vi "Kernel grid search.vi"(8 "Error In":errorcluster, 10 "Grid parameters":T8={"C start"=-5.0, "Gamma start"=-15.0, "C end"=15.0, "C step"=4.0, "K"=10, "Gamma end"=3.0, "Gamma step"=4.0, "random seed"=-1}, 11 "Problem":T1) -> (0 "Error Out":errorcluster, 1 "Kernel":T6, 2 "libsvm":T5, 3 "3D Surface Plot":refnum<class "3D Plot Datatype.lvclass">[](array[class]), 4 "Grid search results":T2)   [LabVIEW 2016]
uses:
  <userlib>/LVLibSVM/LibSVM Sparse/Controls/Grid parameters.ctl
  <userlib>/LVLibSVM/LibSVM Sparse/Controls/Kernel.ctl
  <userlib>/LVLibSVM/LibSVM Sparse/Wrapper API/Controls/svm_kernel_type.ctl
  <userlib>/LVLibSVM/LibSVM Sparse/Controls/Options Training.ctl
  <userlib>/LVLibSVM/LibSVM Sparse/Controls/Parameters C_SVC.ctl
  <vilib>/Math Plots/3D Math Plots/3D Plot/3D Plot Datatype/3D Plot Datatype.lvclass
  <userlib>/LVLibSVM/LibSVM Dense/Wrapper API/Controls/svmdense_problem.ctl
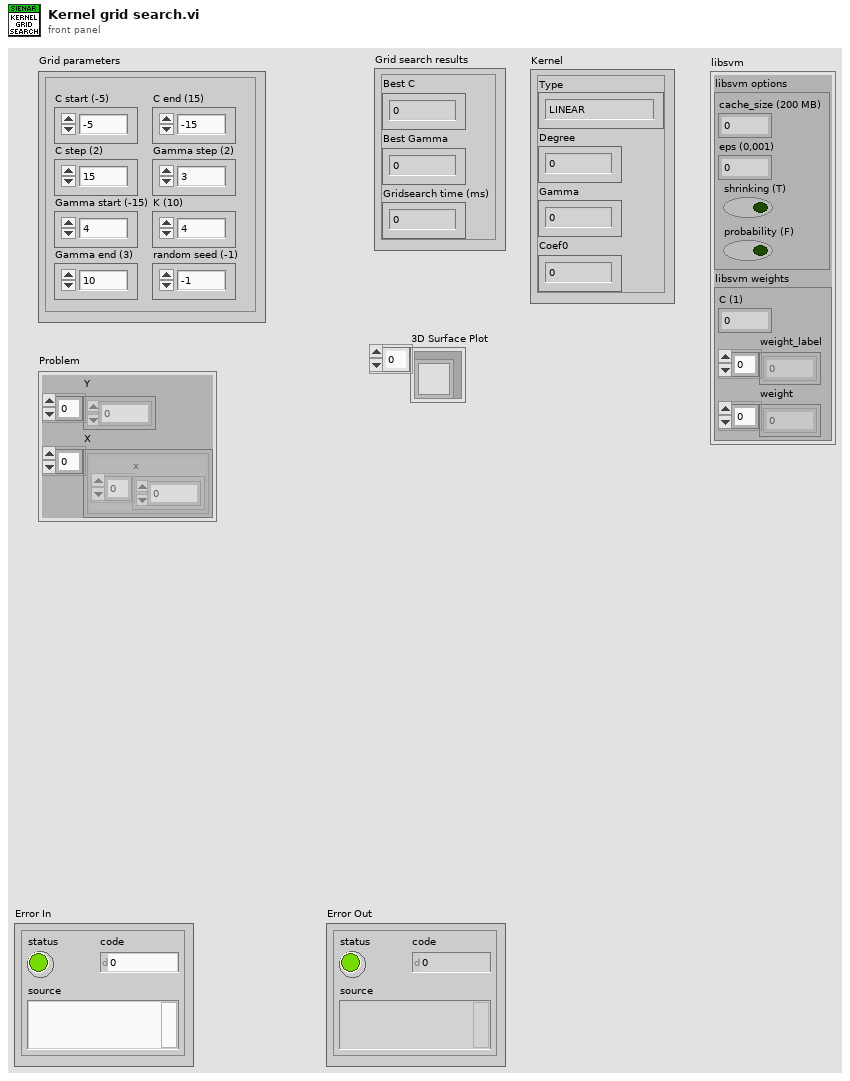
[diagram p1: front panel]
types:
  T1 = typedef "svmdense_problem.ctl" = cluster{"Y":dbl[], "X":cluster{"x":dbl[]}[]}
  T2 = cluster{"Best C":dbl, "Best Gamma":dbl, "Gridsearch time (ms)":u32}
  T3 = typedef "Options Training.ctl" = cluster{"cache_size":dbl, "eps":dbl, "shrinking":bool, "probability":bool}
  T4 = typedef "Parameters C_SVC.ctl" = cluster{"C":dbl, "weight_label":i32[], "weight":dbl[]}
  T5 = cluster{"libsvm options":T3, "libsvm weights":T4}
  T6 = typedef "Kernel.ctl" = cluster{"Type":T7, "Degree":i32, "Gamma":dbl, "Coef0":dbl}
  T7 = typedef "svm_kernel_type.ctl" = enum32{"LINEAR", "POLY", "RBF", "SIGMOID", "PRECOMPUTED"}
  T8 = typedef "Grid parameters.ctl" = cluster{"C start":dbl, "Gamma start":dbl, "C end":dbl, "C step":dbl, "K":i32, "Gamma end":dbl, "Gamma step":dbl, "random seed":i32}
  T9 = typedef "Binary_ConfusionMatrix.ctl" = cluster{"N Total":u32, "N True":u32, "N False":u32, "Overall Rate":dbl, "True Positive":dbl, "False Positive":dbl, "False Negative":dbl, "True Negative":dbl}
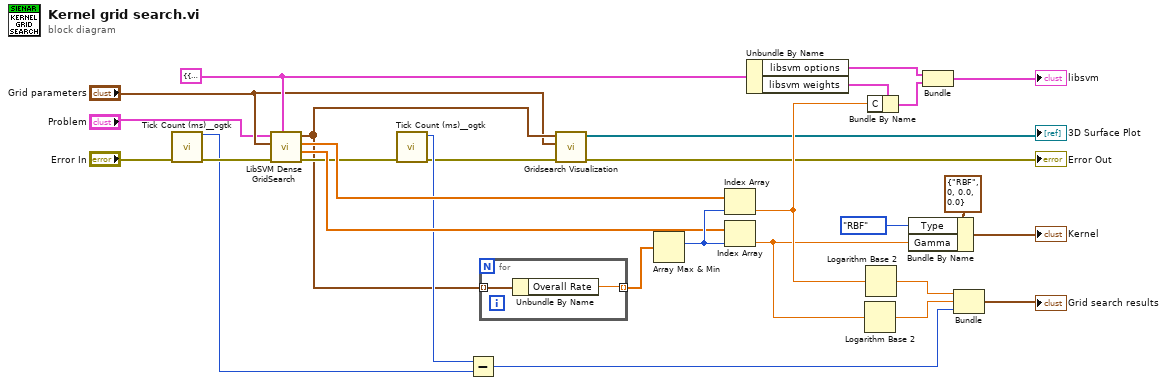
[diagram p0: block diagram]
diagram:
  w22 = T5 {"libsvm options"={"cache_size"=200.0, "eps"=0.001, "shrinking"=TRUE, "probability"=FALSE}, "libsvm weights"={"C"=1.0, "weight_label"=[], "weight"=[]}} ("libsvm")
  n1 = call <userlib>:"Tick Count (ms)__ogtk.vi"("error in (no error)"="Error In") -> ("error out"=w19:errorcluster, "millisecond timer value"=w16:u32)  [unwired: 9 in]
  n2 = call <userlib>:"LibSVM Dense GridSearch.vi"("libsvm"=w22, "error in (no error)"=w19, "Grid parameters"="Grid parameters", "Problem"="Problem") -> ("error out"=w18:errorcluster, "gamma"=w21:dbl[], "C"=w20:dbl[], "Confusion matrices"=w13:T9[])  [unwired: 3 in, 1 out]
  n3 = call <userlib>:"Tick Count (ms)__ogtk.vi"("error in (no error)"=w18) -> ("error out"=w14:errorcluster, "millisecond timer value"=w17:u32)  [unwired: 9 in]
  n4 = Subtract(x=w17, y=w16) -> (x-y=w2:u32)
  n5 = for {
    tunnel: w13 -> [w31] mode=indexing
    tunnel: [w30] -> w29 mode=indexing
    n6 = Unbundle By Name(w31) -> ("Overall Rate"=w30:dbl)
  }
  n7 = call <userlib>:"Gridsearch Visualization.vi"("error in (no error)"=w14, "Grid parameters"="Grid parameters", "Confusion matrices"=w13) -> ("error out"=→"Error Out":errorcluster, "3D Surface Plot"=→"3D Surface Plot":refnum<class "3D Plot Datatype.lvclass">[])  [unwired: 7 in]
  n8 = Array Max & Min(array=w29) -> (max index (indices)=w28:i32)  [unwired: 3 out]
  n9 = Index Array(array=w20, index=w28) -> (element=w24:dbl)
  n10 = Index Array(array=w21, index=w28) -> (element=w23:dbl)
  n11 = Unbundle By Name(w22) -> ("libsvm options"=w5:T3, "libsvm weights"=w27:T4)
  n12 = Logarithm Base 2(1:w23) -> (0:w7:dbl)
  n13 = Logarithm Base 2(1:w24) -> (0:w8:dbl)
  n14 = Bundle By Name(cluster=w27, "C"=w24) -> (w6:T4)
  n15 = Bundle By Name(cluster=T6 {"Type"=enum."RBF", "Degree"=0, "Gamma"=0.0, "Coef0"=0.0} ("Kernel"), "Type"=svm_kernel_type."RBF", "Gamma"=w23) -> (→"Kernel":T6)
  n16 = Bundle("libsvm options"=w5, "libsvm weights"=w6) -> (→"libsvm":T5)  [unwired: 1 in]
  n17 = Bundle(w8, w7, w2) -> (→"Grid search results":cluster{dbl, dbl, u32})  [unwired: 1 in]
